vi "Compile Outgoing Frames.vi"(8 "error in (no error)":errorcluster, 9 "Frame Settings Array":T1[](array[typedef]) {"Signals"."Byte Order" items=["Little Endian", "Big Endian"]; "Signals"."Data Type" items=["Signed", "Unsigned", "IEEE Float"]}, 10 "Refs":T6[](array[typedef]) {"Signal Refs" format="%.0x"}, 11 "Item Ref in":T5 format="%.0x") -> (0 "error out":errorcluster, 1 "output cluster":cluster{"Refs":T3[], "Values":dbl[]} {"Refs"."Data Reference" format="%.0x"}, 2 "Lookup Table":variant, 3 "Item Ref out":T5=18446744073709551615 format="%.0x")   [LabVIEW 2015, in "Diagnostics Addon System Explorer.lvlib"]
uses:
  Diagnostics Addon System Explorer.lvlib
  <vilib>/NI Veristand/Custom Device API/Custom Device Item Ref.ctl
  Types/Frame Signal VS References.ctl
  <vilib>/NI Veristand/Custom Device API/Block Data Reference.ctl
  <vilib>/NI Veristand/Custom Device API/Data Reference.ctl
  Shared/Types/Frame Parameters.ctl
  Shared/Types/Signal Parameters.ctl
  <vilib>/NI Veristand/Custom Device API/Data Access Type.ctl
  Shared/Types/Datatable Lookup Positions.ctl
  Shared/Diagnostics Addon Shared.lvlib
  <vilib>/NI Veristand/Custom Device API/Custom Device API.lvlib
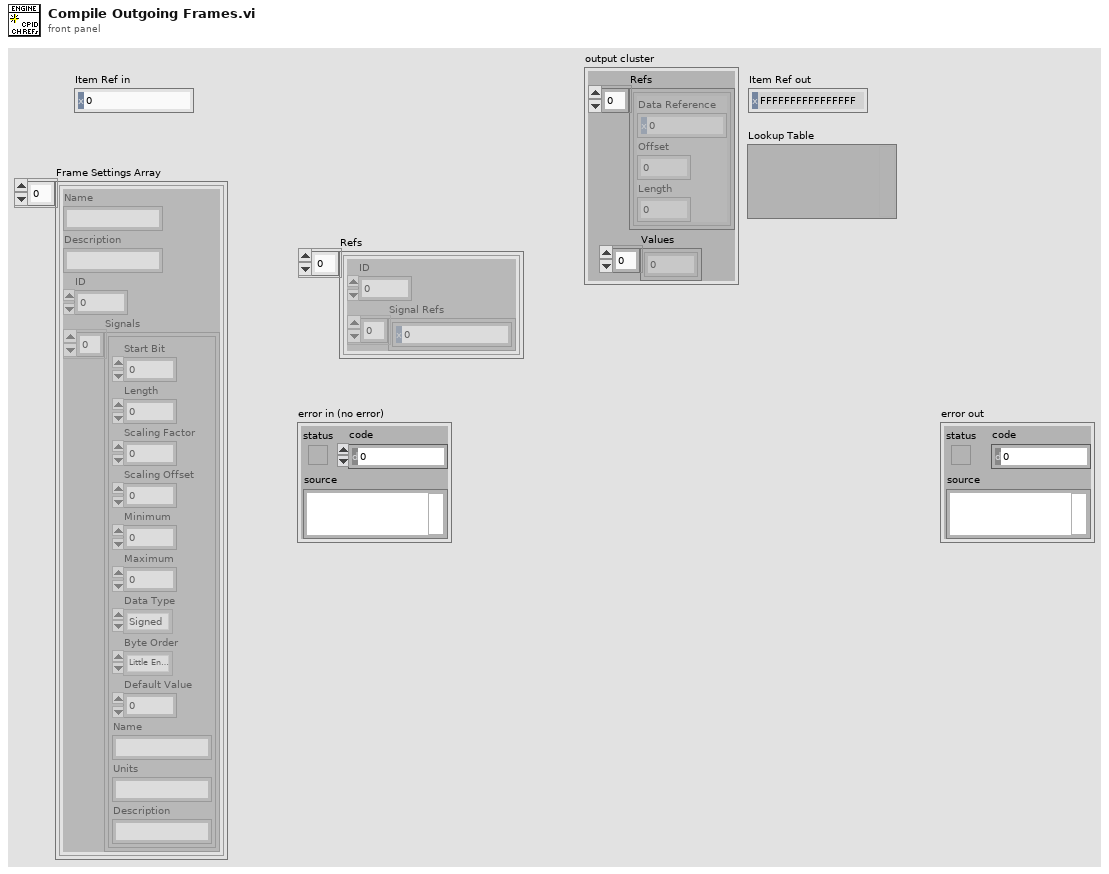
[diagram p1: front panel]
types:
  T1 = typedef "Diagnostics Addon Shared.lvlib/Frame Parameters.ctl" = cluster{"Name":string, "Description":string, "ID":u32, "Signals":T2[]}
  T2 = typedef "Diagnostics Addon Shared.lvlib/Signal Parameters.ctl" = cluster{"Start Bit":u8, "Length":u8, "Scaling Factor":dbl, "Scaling Offset":dbl, "Minimum":dbl, "Maximum":dbl, "Data Type":u32, "Byte Order":u32, "Default Value":dbl, "Name":string, "Units":string, "Description":string}
  T3 = typedef "Custom Device API.lvlib/Block Data Reference.ctl" = cluster{"Data Reference":T4, "Offset":u64, "Length":u64}
  T4 = typedef "Custom Device API.lvlib/Data Reference.ctl" = i32
  T5 = typedef "Custom Device API.lvlib/Custom Device Item Ref.ctl" = u64
  T6 = typedef "Diagnostics Addon System Explorer.lvlib/Frame Signal VS References.ctl" = cluster{"ID":u32, "Signal Refs":T5[]}
  T7 = typedef "Custom Device API.lvlib/Data Access Type.ctl" = enum16{"Read", "Write"}
  T8 = typedef "Diagnostics Addon Shared.lvlib/Datatable Lookup Positions.ctl" = cluster{"Offset":i32, "Length":i32, "ByteLength":u16}
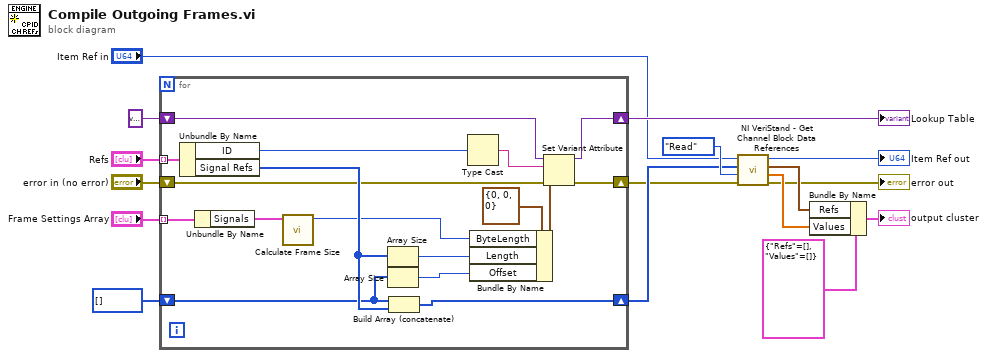
[diagram p0: block diagram]
diagram:
  n1 = for {
    tunnel: "Refs" -> [w25] mode=indexing
    shift-right: [w26] -> w13
    shift-left: variant -> [w30]
    shift-right: [w28] -> w5
    shift-left: "error in (no error)" -> [w21]
    shift-right: [w24] -> w10
    shift-left: T5[] [] -> [w22]
    tunnel: "Frame Settings Array" -> [w20] mode=indexing
    n2 = Unbundle By Name(w25) -> ("ID"=w17:u32, "Signal Refs"=w23:T5[])
    n3 = Unbundle By Name(w20) -> ("Signals"=w19:T2[])
    n4 = call "Calculate Frame Size.vi"("Parameters"=w19) -> ("Bytes"=w18:u16)  [unwired: 10 in]
    n5 = Array Size(array=w23) -> (size(s)=w33:i32)
    n6 = Array Size(array=w22) -> (size(s)=w29:i32)
    n7 = Build Array (concatenate)(w22, w23) -> (w24:T5[])
    n8 = Type Cast(x=w17) -> (*(type *) &x=w27:string)  [unwired: 1 in]
    n9 = Bundle By Name(cluster=T8 {"Offset"=0, "Length"=0, "ByteLength"=0}, "ByteLength"=w18, "Length"=w33, "Offset"=w29) -> (w31:T8)
    n10 = Set Variant Attribute(Variant=w30, name=w27, value=w31, error in=w21) -> (Variant out=w26:variant, error out=w28:errorcluster)  [unwired: 1 out]
  }
  "Lookup Table" <- w13
  n11 = call <vilib>:"NI VeriStand - Get Channel Block Data References.vi"("error in (no error)"=w5, "Access"=Data_Access_Type."Read", "Channel Refs"=w10, "Device Ref in"="Item Ref in") -> ("error out"=→"error out":errorcluster, "Values Array"=w6:dbl[], "Block Data Refs"=w7:T3[], "Device Ref out"=→"Item Ref out":T5)  [unwired: 4 in]
  n12 = Bundle By Name(cluster=cluster{"Refs":T3[], "Values":dbl[]} {"Refs"=[], "Values"=[]} ("Pairs"), "Refs"=w7, "Values"=w6) -> (→"output cluster":cluster{"Refs":T3[], "Values":dbl[]})
